vi "维持时间.vi"(7 "refnum":T1 caption="引用句柄", 10 "测试人员":string, 11 "错误输入（无错误）":errorcluster) -> (2 "维持时间":T2={"测试参数"={"读取电压(V)"=0.0, "极限电流(mA)"=0.0}, "时序参数"={"测试时间(s)"=0.0, "读取间隔(ms)"=0.0, "nplc"=0.001, "时序优先"=FALSE}} {"时序参数"."nplc" min=0.001; "测试参数"."极限电流(mA)" min=0.0 max=3000.0; "测试参数"."读取电压(V)" min=-40.0 max=40.0}, 3 "错误输出":errorcluster, 5 "refnum out":T1 caption="引用句柄输出")   [LabVIEW 2020]
uses:
  <vilib>/Utility/config.llb/NI_LVConfig.lvlib
  <vilib>/Utility/config.llb/Read Key (String).vi
  <vilib>/Utility/config.llb/Config Data RefNum.ctl
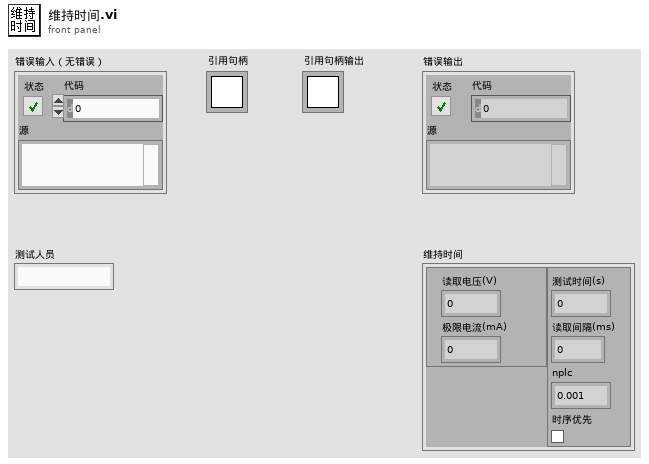
[diagram p1: front panel]
types:
  T1 = typedef "NI_LVConfig.lvlib/Config Data RefNum.ctl" = refnum<k1>
  T2 = typedef "维持时间.ctl" = cluster{"测试参数":cluster{"读取电压(V)":dbl, "极限电流(mA)":dbl}, "时序参数":cluster{"测试时间(s)":dbl, "读取间隔(ms)":dbl, "nplc":dbl, "时序优先":bool}}
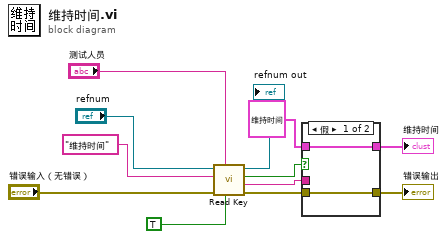
[diagram p0: block diagram]
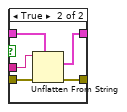
[diagram p2: hidden frame]
diagram:
  n1 = call-poly <vilib>:"Read Key.vi"("read raw string? (F)"=TRUE, "section"="测试人员", "error in (no error)"="错误输入（无错误）", "key"="维持时间", "refnum"="refnum") -> ("error out"=w3:errorcluster, "value"=w8:string, "found?"=w7:bool, "refnum out"=→"refnum out":T1)  [unwired: 3 in]
  n2 = case shown="假" w7 {
    tunnel: w8 -> [_ w19]
    tunnel: T2 {"测试参数"={"读取电压(V)"=1.0, "极限电流(mA)"=1.0}, "时序参数"={"测试时间(s)"=10.0, "读取间隔(ms)"=10.0, "nplc"=1.0, "时序优先"=FALSE}} ("维持时间") -> [w14 w18]
    tunnel: [w14 w17] -> w5
    tunnel: [w13 w16] -> w4
    tunnel: w3 -> [w13 w15]
    frame False {
    }
    frame True {
      n3 = Unflatten From String(type=w18, binary string=w19, error in (no error)=w15) -> (value=w17:T2, error out=w16:errorcluster)  [unwired: 2 in, 1 out]
    }
  }
  "错误输出" <- w4
  "维持时间" <- w5
